vi "02 - Demonstration - Event Queue Decoupled from Generation.vi"() -> ()   [LabVIEW 2012]
panel:
  out "Chart of memory used by this VI (appx)":sgl(graph) caption="Memory used by this VI (MB, appx)"
  in  "Suspend B":bool
  in  "Suspend A":bool
  in  "Kill the Messenger":bool
  in  "Register B":bool
  in  "Unregister B":bool
  in  "Unregister A":bool
  in  "Register A":bool
  out "Messages Sent":i32 format="Messages sent: %d"
  in  "stop":bool
  # "Subscriber A"
  # "Subscriber B"
  # "Demonstrations\n1. Run the VI, noting how \"Messages Sent\" continually increases yet \"Memory used by this VI\" is not. Published messages with no subscribers 'vanish'\n\n2. Register A. Suspend A. Unregister A. Repeat, using B, noting identical behaviors\n\n3. Register A, then B. (Note: slope is unchanged). Suspend A, then B. Now, Unregister B (Note: plateau drops to level when B was first registered.)\n\n4. Register A. Now, 'Kill the Messenger'. Note how memory plateaus, with A no longer receiving messages, yet retaining existing messages."
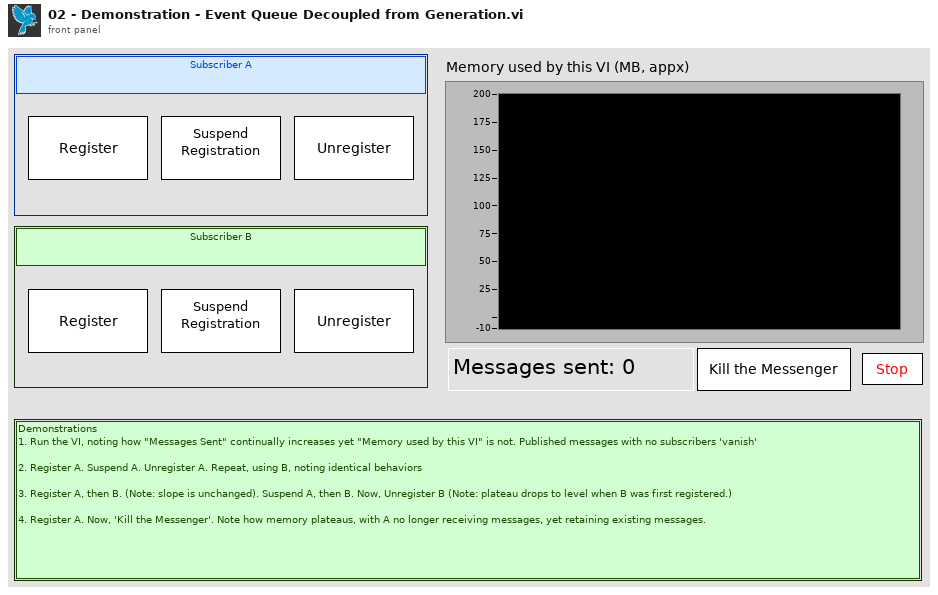
[diagram p1: front panel]
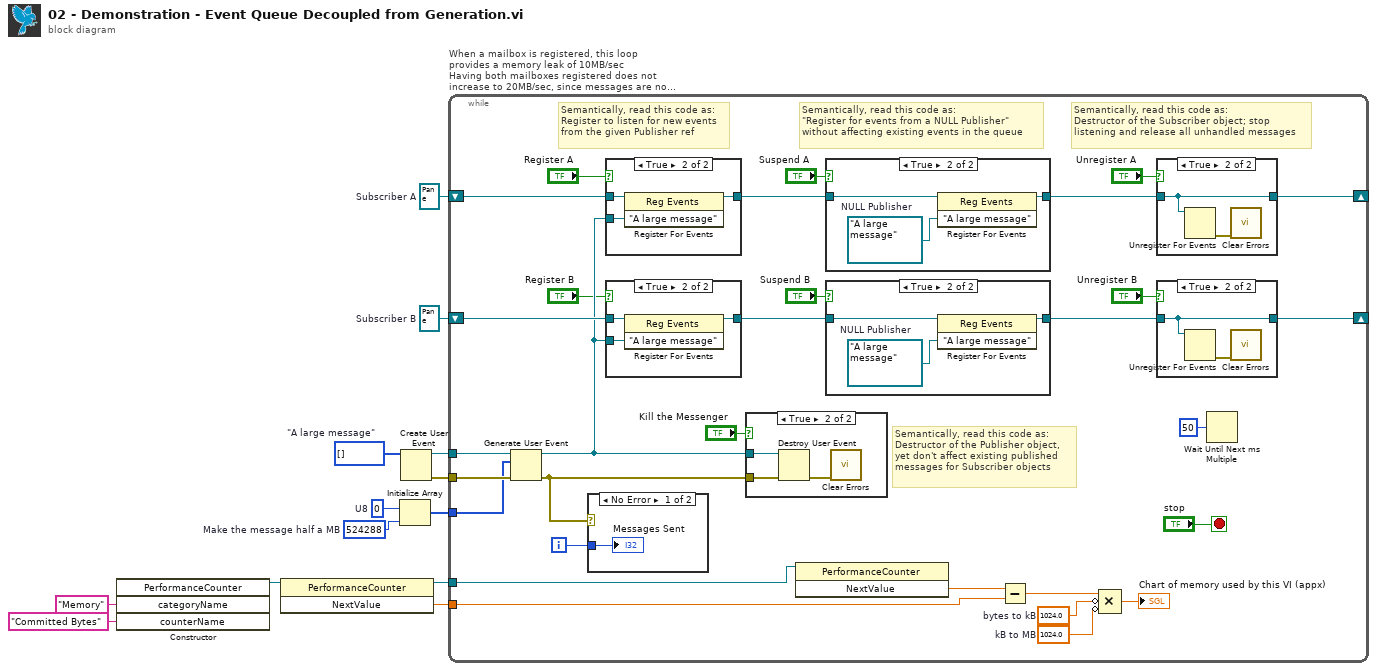
[diagram p0: block diagram]
diagram:
  w6 = refnum<event-registration> refnum  # Subscriber A
  w7 = refnum<event-registration> refnum  # Subscriber B
  w8 = u8[] []  # "A large message"
  w12 = 524288  # Make the message half a MB
  w13 = u8 0  # U8
  n1 = constructor class="PerformanceCounter"("categoryName"="Memory", "counterName"="Committed Bytes") -> (reference out=w3:refnum<k24>)  [unwired: 3 in, 4 out]
  n2 = invoke class="PerformanceCounter" method="NextValue"(reference=w3) -> (reference out=w2:refnum<k24>, "NextValue"=w1:sgl)  [unwired: 2 in, 1 out]
  n3 = Initialize Array(w13, w12) -> (w9:u8[])
  n4 = Create User Event(user event datatype=w8) -> (user event=w10:refnum<user-event>, error out=w11:errorcluster)  [unwired: 1 in]
  n5 = while "When a mailbox is registered, this loop provides a memory leak of 10MB/sec\nHaving both mailboxes registered does not increase to 20MB/sec, since messages are not duplicated til handled." {
    tunnel: w11 -> [w42]
    tunnel: w10 -> [w43]
    tunnel: w9 -> [w40]
    shift-right: [w35] -> _
    shift-left: w7 -> [w38]
    shift-right: [w36] -> _
    shift-left: w6 -> [w37]
    tunnel: w2 -> [w20]
    tunnel: w1 -> [w17]
    i -> [w31]
    stop <- "stop" stop-if-true
    w18 = sgl 1024.0  # kB to MB
    w19 = sgl 1024.0  # bytes to kB
    # "Semantically, read this code as:\nDestructor of the Publisher object,\nyet don't affect existing published\nmessages for Subscriber objects"
    # "Semantically, read this code as:\nRegister to listen for new events\nfrom the given Publisher ref"
    # "Semantically, read this code as:\nDestructor of the Subscriber object; stop\nlistening and release all unhandled messages"
    # "Semantically, read this code as:\n\"Register for events from a NULL Publisher\"\nwithout affecting existing events in the queue"
    n6 = Generate User Event(user event=w43, event data cluster=w40, error in=w42) -> (user event out=w33:refnum<user-event>, error out=w32:errorcluster)
    n7 = case shown="No Error" w32 {
      tunnel: w31 -> [w52 _]
      frame No Error {
        "Messages Sent" <- w52
      }
      frame Error {
      }
    }
    n8 = case shown="True" "Register A" {
      tunnel: w33 -> [_ w65]
      tunnel: w37 -> [w62 w64]
      tunnel: [w62 w63] -> w28
      frame False {
      }
      frame True {
        n9 = register-events(reference=w64, w65) -> (reference out=w63:refnum<event-registration>)  [unwired: 1 in, 1 out]
      }
    }
    n10 = case shown="True" "Register B" {
      tunnel: w33 -> [_ w69]
      tunnel: w38 -> [w66 w68]
      tunnel: [w66 w67] -> w30
      frame False {
      }
      frame True {
        n11 = register-events(reference=w68, w69) -> (reference out=w67:refnum<event-registration>)  [unwired: 1 in, 1 out]
      }
    }
    n12 = case shown="True" "Kill the Messenger" {
      tunnel: w33 -> [_ w55]
      tunnel: w32 -> [_ w54]
      frame False {
      }
      frame True {
        n13 = Destroy User Event(user event=w55, error in=w54) -> (error out=w53:errorcluster)
        n14 = call <vilib>:"Clear Errors.vi"("error in (no error)"=w53) -> ()  [unwired: 6 in, 1 out]
      }
    }
    n15 = invoke class="PerformanceCounter" method="NextValue"(reference=w20) -> ("NextValue"=w16:sgl)  [unwired: 2 in, 2 out]
    n16 = case shown="True" "Suspend A" {
      tunnel: w28 -> [w44 w47]
      tunnel: [w44 w46] -> w27
      frame False {
      }
      frame True {
        w45 = refnum<user-event> refnum  # NULL Publisher
        n17 = register-events(reference=w47, w45) -> (reference out=w46:refnum<event-registration>)  [unwired: 1 in, 1 out]
      }
    }
    n18 = case shown="True" "Suspend B" {
      tunnel: w30 -> [w48 w51]
      tunnel: [w48 w50] -> w29
      frame False {
      }
      frame True {
        w49 = refnum<user-event> refnum  # NULL Publisher
        n19 = register-events(reference=w51, w49) -> (reference out=w50:refnum<event-registration>)  [unwired: 1 in, 1 out]
      }
    }
    n20 = Subtract(x=w16, y=w17) -> (x-y=w15:sgl)
    n21 = Compound Arithmetic op=MULTIPLY(w15, invert w19, invert w18) -> (→"Chart of memory used by this VI (appx)":sgl)
    n22 = case shown="True" "Unregister A" {
      tunnel: w27 -> [w59 w61]
      tunnel: [w59 w61] -> w36
      frame False {
      }
      frame True {
        n23 = Unregister For Events(event registration refnum=w61) -> (error out=w60:errorcluster)  [unwired: 1 in]
        n24 = call <vilib>:"Clear Errors.vi"("error in (no error)"=w60) -> ()  [unwired: 6 in, 1 out]
      }
    }
    n25 = case shown="True" "Unregister B" {
      tunnel: w29 -> [w56 w58]
      tunnel: [w56 w58] -> w35
      frame False {
      }
      frame True {
        n26 = Unregister For Events(event registration refnum=w58) -> (error out=w57:errorcluster)  [unwired: 1 in]
        n27 = call <vilib>:"Clear Errors.vi"("error in (no error)"=w57) -> ()  [unwired: 6 in, 1 out]
      }
    }
    n28 = Wait Until Next ms Multiple(millisecond multiple=u32 50) -> ()  [unwired: 1 out]
  }
